vi "LVClass_Camera set TimeOUT.vi"(0 "Camera in":refnum<class "Camera.lvclass">, 5 "timeout":u32, 11 "error in (no error)":errorcluster) -> (4 "Camera out":refnum<class "Camera.lvclass">, 15 "error out":errorcluster)   [LabVIEW 2020, in "Camera.lvclass"]
doc: "Set Camera time out value.\n\n<B>CameraIn</B> : Camera object.\n<B>CameraOut</B> : Camera object.\n<B>TimeOut</B> : Time out value (ms)."
uses:
  Camera.lvclass
  Camera.lvclass/Camera.ctl
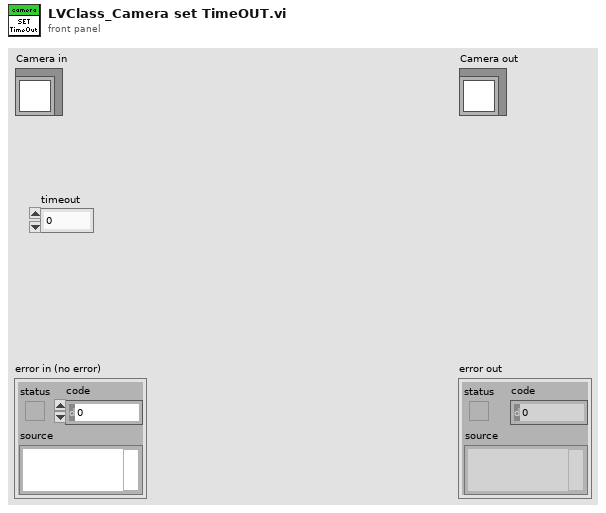
[diagram p1: front panel]
types:
  T1 = typedef "ClassID.ctl" = i64
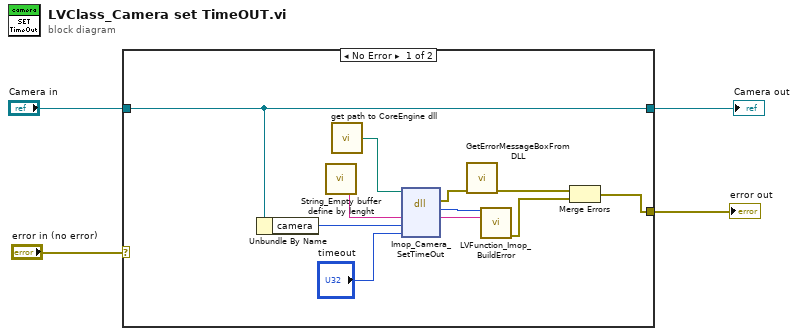
[diagram p0: block diagram]
diagram:
  n1 = case shown="No Error" "error in (no error)" {
    selector: "error in (no error)" -> [_ w17]
    tunnel: [w5 w17] -> w3
    tunnel: [w11 w16] -> w1
    tunnel: "Camera in" -> [w11 w16]
    frame No Error {
      n2 = Unbundle By Name(w11) -> ("camera"=w12:T1)
      n3 = call "String_Empty buffer define by lenght.vi"() -> ("Empty buffer"=w15:string)  [unwired: 1 in]
      n4 = call "get path to CoreEngine dll.vi"() -> ("path to wavekit library"=w9:path)  [unwired: 14 in, 1 out]
      n5 = dll-call lib="D:/soft/HASO_v3/SVN_trunk/ImOpCoreEngine4_LV2011/DLLs/c_interface_vc100.dll" fn="Imop_Camera_SetTimeOut"(path in=w9, "message"=w15, "camera"=w12, "timeout"="timeout") -> (error out=w8:errorcluster, "return type"=w14:i32, "message"=w13:string)  [unwired: 4 in, 1 out]
      n6 = call "GetErrorMessageBoxFromDLL.vi"("error IN"=w8) -> ("error OUT"=w7:errorcluster)  [unwired: 10 in]
      n7 = call "LVFunction_Imop_BuildError.vi"("code"=w14, "String to Prepend to source (\"\")"=w13) -> ("error out"=w6:errorcluster)  [unwired: 13 in]
      n8 = Merge Errors(w7, w6) -> (w5:errorcluster)
    }
    frame Error {
    }
  }
  "error out" <- w3
  "Camera out" <- w1
